vi "G2CPU Line Indexes To Coordinates.vi"(4 "Auto Release Points of Interest on Lines (Enabled)":bool=TRUE, 6 "Auto Release Line Indexers":T1={"Auto Release Line Indexers (Enabled)"=TRUE, "Auto Release Keys (Enabled)"=TRUE}, 8 "error in (no error)":errorcluster, 10 "Line Indexers":T3, 11 "Point of Interest on Lines":refnum<class "1D Array f32.lvclass">) -> (0 "error out":errorcluster, 3 "Coordinates Out":T2)   [LabVIEW 2020, in "G2CPU Line Profile.lvlib"]
doc: "Transform locations on the line profiles to coordinates on the image."
uses:
  G2CPU Line Profile.lvlib
  <vilib>/Natan Biesmans/G2CPU GPU and CPU HPC Toolkit/G2CPU Libraries/Arrays/1DArray/f32/1D Array f32.lvclass
  C:/Program Files/National Instruments/LabVIEW 2025/vi.lib/Natan Biesmans/G2CPU GPU and CPU HPC Toolkit/G2CPU Libraries/Arrays/Array/Array Prototype.lvclass
  <vilib>/Natan Biesmans/G2CPU GPU and CPU HPC Toolkit/G2CPU Libraries/Arrays/2DArray/f32/2D Array f32.lvclass
  <vilib>/Natan Biesmans/G2CPU GPU and CPU HPC Toolkit/G2CPU Libraries/Arrays/2DArray/u32/2D Array u32.lvclass
  <vilib>/Natan Biesmans/G2CPU GPU and CPU HPC Toolkit/G2CPU Libraries/Arrays/1DArray/u32/1D Array u32.lvclass
  <vilib>/Natan Biesmans/G2CPU GPU and CPU HPC Toolkit/G2CPU Libraries/Assignment and indexing/Indexers/G2CPU Indexers.lvclass/G2CPU Indexers.ctl
  <vilib>/Natan Biesmans/G2CPU GPU and CPU HPC Toolkit/G2CPU Libraries/Arrays/Array/Array Prototype.lvclass/Array Prototype.ctl
  6af54969-3e89-456c-a305-a66f3c4e0a45.vi
  a8428e5e-e638-4b8f-97b1-1dfa639c029e.vi
  cd2e55c8-9bfa-4798-9cad-c9068625d012.vi
  0cc7a96f-73a6-40f4-8601-915cc3ecb668.vi
  a76dfa27-2fb7-4ce4-a6bc-f21a5bf6cb57.vi
  af729f83-0425-4644-a175-0b2d98955893.vi
  2fdfb383-b567-4129-8a88-0dd6299b1c5c.vi
  16f8b6bd-ee5f-4b77-ad5a-b16a773401c6.vi
  240874d8-aa58-4a67-9154-73ea1cbf8ba2.vi
  4e0f6f57-f7b3-4ae1-a782-0e163578409f.vi
  bb7fe687-00b1-4455-be70-867d530c61a9.vi
  d411a91c-f4fd-4c23-b328-89003a8b9fa9.vi
  0eb13b9f-5540-4dae-96e9-dbe1488eafb0.vi
  b1fa1afe-a8d8-4705-ab8c-01af7051f9a8.vi
  24612132-8e46-4228-9c8d-2f2d4fc0b450.vi
  a8f317de-a3ee-4dc2-bb18-38ac143a68e4.vi
  788818c2-d318-43e7-b0fc-c88029d63408.vi
  b03dc83b-e216-4518-af22-f4bd8ac76618.vi
  <vilib>/Natan Biesmans/G2CPU GPU and CPU HPC Toolkit/G2CPU Libraries/Assignment and indexing/Indexers/G2CPU Create Indexer.vi
  <vilib>/Natan Biesmans/G2CPU GPU and CPU HPC Toolkit/G2CPU Libraries/Assignment and indexing/Indexers/G2CPU Add Sequencer.vi
  6af54969-3e89-456c-a305-a66f3c4e0a45.vi/4a09c0ae-6cb4-4568-a5ad-7980d18d146b.vi
  6af54969-3e89-456c-a305-a66f3c4e0a45.vi/9f568e59-a541-4346-a017-6cb4bc957f61.vi
  6af54969-3e89-456c-a305-a66f3c4e0a45.vi/c972bab7-bbaf-49da-9265-270ac06aa9b1.vi
  6af54969-3e89-456c-a305-a66f3c4e0a45.vi/693b35e6-7886-4543-b6bf-58b41be5c5ca.vi
  6af54969-3e89-456c-a305-a66f3c4e0a45.vi/9ef54e8b-cde1-4413-ad7f-8efe3ab0591f.vi
  6af54969-3e89-456c-a305-a66f3c4e0a45.vi/d54d4b2e-96c7-4097-8c0a-576c6fb591be.vi
  <vilib>/Natan Biesmans/G2CPU GPU and CPU HPC Toolkit/G2CPU Libraries/Arrays/Array/G2CPU Get Array Pointer.vi
  a8428e5e-e638-4b8f-97b1-1dfa639c029e.vi/cf27cc0d-1fb9-4e2f-ac40-7e8a0db6b27f.vi
  a8428e5e-e638-4b8f-97b1-1dfa639c029e.vi/1874d702-7e82-49f0-9e52-8a9dc00bddc1.vi
  a8428e5e-e638-4b8f-97b1-1dfa639c029e.vi/d603c635-5557-46f9-9702-9944444483a4.vi
  cd2e55c8-9bfa-4798-9cad-c9068625d012.vi/2cbae9c5-d993-4013-91e6-67de96abb5a0.vi
  cd2e55c8-9bfa-4798-9cad-c9068625d012.vi/df7b902d-6356-419a-b5d5-2ac54df1e506.vi
  0cc7a96f-73a6-40f4-8601-915cc3ecb668.vi/6197f869-f6d4-49b3-9b2c-cc979b422c2e.vi
  0cc7a96f-73a6-40f4-8601-915cc3ecb668.vi/a7e86dbb-b4c0-485c-89c5-522e60ee265c.vi
  a76dfa27-2fb7-4ce4-a6bc-f21a5bf6cb57.vi/5793b77b-c002-4ebf-9075-685617c95341.vi
  a76dfa27-2fb7-4ce4-a6bc-f21a5bf6cb57.vi/2ed3ef86-c00d-4d71-b84c-20267a6dfcf9.vi
  af729f83-0425-4644-a175-0b2d98955893.vi/4181b2af-0669-475f-8228-b34a8d51a6f4.vi
  2fdfb383-b567-4129-8a88-0dd6299b1c5c.vi/e7247370-a01f-465a-ac0e-4dfefcb1bb87.vi
  2fdfb383-b567-4129-8a88-0dd6299b1c5c.vi/345e91f0-9a5e-4de4-af9c-133346717e4a.vi
  16f8b6bd-ee5f-4b77-ad5a-b16a773401c6.vi/7467a0f1-0650-4e63-b635-b3d2b2ec9a4e.vi
  16f8b6bd-ee5f-4b77-ad5a-b16a773401c6.vi/8ee11bc3-5ef5-497e-97f0-8db2b3aaa149.vi
  16f8b6bd-ee5f-4b77-ad5a-b16a773401c6.vi/c7af9698-5e3c-4e11-95da-3024075b67d2.vi
  240874d8-aa58-4a67-9154-73ea1cbf8ba2.vi/2e03f477-51b7-4ba0-bb4f-4f838f6557e6.vi
  240874d8-aa58-4a67-9154-73ea1cbf8ba2.vi/125d45d4-836b-469d-8a4a-6adb452f866d.vi
  240874d8-aa58-4a67-9154-73ea1cbf8ba2.vi/8038e9ed-2e71-4568-91ba-0d873494c5ed.vi
  4e0f6f57-f7b3-4ae1-a782-0e163578409f.vi/9d769ba4-bbb4-4eb6-9175-95d7d139327c.vi
  4e0f6f57-f7b3-4ae1-a782-0e163578409f.vi/8bfea9e7-a130-4d69-b32e-15c58d17157f.vi
  4e0f6f57-f7b3-4ae1-a782-0e163578409f.vi/25f1b8bb-c437-45f4-b6eb-f3e32cc20aa5.vi
  4e0f6f57-f7b3-4ae1-a782-0e163578409f.vi/309f54b5-9a40-4a1d-900d-2d620fefb202.vi
  bb7fe687-00b1-4455-be70-867d530c61a9.vi/bb516b05-0a1d-45df-9cb0-c772dcc1833e.vi
  bb7fe687-00b1-4455-be70-867d530c61a9.vi/2071ba82-ee09-44c2-9784-3e752811cb07.vi
  bb7fe687-00b1-4455-be70-867d530c61a9.vi/c68a08d6-cad3-47fe-810c-4c138e8e5bf7.vi
  bb7fe687-00b1-4455-be70-867d530c61a9.vi/599fcc89-82aa-4e20-b9df-949478d910a7.vi
  d411a91c-f4fd-4c23-b328-89003a8b9fa9.vi/ce577589-e75d-42be-a3c5-f5395febe2a6.vi
  d411a91c-f4fd-4c23-b328-89003a8b9fa9.vi/d13051aa-bce5-446f-b44f-e7ab7cfb1f03.vi
  d411a91c-f4fd-4c23-b328-89003a8b9fa9.vi/ca2a5711-2ea0-41ce-865a-169a0e3bc9ca.vi
  0eb13b9f-5540-4dae-96e9-dbe1488eafb0.vi/f4654d05-beb0-4753-bab7-24376daae318.vi
  0eb13b9f-5540-4dae-96e9-dbe1488eafb0.vi/a2f9e1c9-c94e-4cd6-9432-cf54c3ac582a.vi
  b1fa1afe-a8d8-4705-ab8c-01af7051f9a8.vi/d8f9d983-4edf-44a2-8364-f00f0b470774.vi
  b1fa1afe-a8d8-4705-ab8c-01af7051f9a8.vi/83167447-a0f5-45d9-a71d-4def8f50970d.vi
  24612132-8e46-4228-9c8d-2f2d4fc0b450.vi/cfed8f62-9c64-4dab-912e-5e7c21cb720b.vi
  a8f317de-a3ee-4dc2-bb18-38ac143a68e4.vi/d8f9d983-4edf-44a2-8364-f00f0b470774.vi
  a8f317de-a3ee-4dc2-bb18-38ac143a68e4.vi/83167447-a0f5-45d9-a71d-4def8f50970d.vi
  788818c2-d318-43e7-b0fc-c88029d63408.vi/cfed8f62-9c64-4dab-912e-5e7c21cb720b.vi
  b03dc83b-e216-4518-af22-f4bd8ac76618.vi/d8f9d983-4edf-44a2-8364-f00f0b470774.vi
  b03dc83b-e216-4518-af22-f4bd8ac76618.vi/83167447-a0f5-45d9-a71d-4def8f50970d.vi
  <vilib>/Natan Biesmans/G2CPU GPU and CPU HPC Toolkit/G2CPU Libraries/Assignment and indexing/Indexers/G2CPU Get indexers Pointer.vi
  a8428e5e-e638-4b8f-97b1-1dfa639c029e.vi/cf27cc0d-1fb9-4e2f-ac40-7e8a0db6b27f.vi/3e802c67-fb96-46a3-ae13-4994a8508b4f.vi
  a8428e5e-e638-4b8f-97b1-1dfa639c029e.vi/cf27cc0d-1fb9-4e2f-ac40-7e8a0db6b27f.vi/5a50fc67-79e7-4972-80c2-92243cd53dd4.vi
  a8428e5e-e638-4b8f-97b1-1dfa639c029e.vi/cf27cc0d-1fb9-4e2f-ac40-7e8a0db6b27f.vi/4b7910ad-0c4a-46e4-b1b3-c9721aeaa91e.vi
  a8428e5e-e638-4b8f-97b1-1dfa639c029e.vi/1874d702-7e82-49f0-9e52-8a9dc00bddc1.vi/77c7badc-ed81-4514-99c1-20d37f4e5ecc.vi
  a8428e5e-e638-4b8f-97b1-1dfa639c029e.vi/1874d702-7e82-49f0-9e52-8a9dc00bddc1.vi/eb76fa01-6782-47b4-b34f-9eb474c9cc78.vi
  <vilib>/Natan Biesmans/G2CPU GPU and CPU HPC Toolkit/ArrayFire Driver/VIs/Run as Multi Device.vi
  a8428e5e-e638-4b8f-97b1-1dfa639c029e.vi/d603c635-5557-46f9-9702-9944444483a4.vi/730f6c57-5c0b-4ee9-b61e-75067b25222b.vi
  a8428e5e-e638-4b8f-97b1-1dfa639c029e.vi/d603c635-5557-46f9-9702-9944444483a4.vi/096b8799-7810-404e-baca-ba9279cec4bd.vi
  a8428e5e-e638-4b8f-97b1-1dfa639c029e.vi/d603c635-5557-46f9-9702-9944444483a4.vi/0f1a5a47-bcc5-4796-ac31-8dfcfbc0d7d1.vi
  a8428e5e-e638-4b8f-97b1-1dfa639c029e.vi/d603c635-5557-46f9-9702-9944444483a4.vi/89f12e17-3330-4b72-ad8f-8dd636660732.vi
  cd2e55c8-9bfa-4798-9cad-c9068625d012.vi/df7b902d-6356-419a-b5d5-2ac54df1e506.vi/6058dca8-195d-4566-b47b-6d6a1c5af61f.vi
  0cc7a96f-73a6-40f4-8601-915cc3ecb668.vi/6197f869-f6d4-49b3-9b2c-cc979b422c2e.vi/3e802c67-fb96-46a3-ae13-4994a8508b4f.vi
  0cc7a96f-73a6-40f4-8601-915cc3ecb668.vi/6197f869-f6d4-49b3-9b2c-cc979b422c2e.vi/5a50fc67-79e7-4972-80c2-92243cd53dd4.vi
  0cc7a96f-73a6-40f4-8601-915cc3ecb668.vi/6197f869-f6d4-49b3-9b2c-cc979b422c2e.vi/4b7910ad-0c4a-46e4-b1b3-c9721aeaa91e.vi
  0cc7a96f-73a6-40f4-8601-915cc3ecb668.vi/a7e86dbb-b4c0-485c-89c5-522e60ee265c.vi/730f6c57-5c0b-4ee9-b61e-75067b25222b.vi
  0cc7a96f-73a6-40f4-8601-915cc3ecb668.vi/a7e86dbb-b4c0-485c-89c5-522e60ee265c.vi/096b8799-7810-404e-baca-ba9279cec4bd.vi
  0cc7a96f-73a6-40f4-8601-915cc3ecb668.vi/a7e86dbb-b4c0-485c-89c5-522e60ee265c.vi/0f1a5a47-bcc5-4796-ac31-8dfcfbc0d7d1.vi
  0cc7a96f-73a6-40f4-8601-915cc3ecb668.vi/a7e86dbb-b4c0-485c-89c5-522e60ee265c.vi/89f12e17-3330-4b72-ad8f-8dd636660732.vi
  a76dfa27-2fb7-4ce4-a6bc-f21a5bf6cb57.vi/5793b77b-c002-4ebf-9075-685617c95341.vi/3e802c67-fb96-46a3-ae13-4994a8508b4f.vi
  a76dfa27-2fb7-4ce4-a6bc-f21a5bf6cb57.vi/5793b77b-c002-4ebf-9075-685617c95341.vi/5a50fc67-79e7-4972-80c2-92243cd53dd4.vi
  a76dfa27-2fb7-4ce4-a6bc-f21a5bf6cb57.vi/2ed3ef86-c00d-4d71-b84c-20267a6dfcf9.vi/730f6c57-5c0b-4ee9-b61e-75067b25222b.vi
  a76dfa27-2fb7-4ce4-a6bc-f21a5bf6cb57.vi/2ed3ef86-c00d-4d71-b84c-20267a6dfcf9.vi/096b8799-7810-404e-baca-ba9279cec4bd.vi
  a76dfa27-2fb7-4ce4-a6bc-f21a5bf6cb57.vi/2ed3ef86-c00d-4d71-b84c-20267a6dfcf9.vi/0f1a5a47-bcc5-4796-ac31-8dfcfbc0d7d1.vi
  a76dfa27-2fb7-4ce4-a6bc-f21a5bf6cb57.vi/2ed3ef86-c00d-4d71-b84c-20267a6dfcf9.vi/89f12e17-3330-4b72-ad8f-8dd636660732.vi
  240874d8-aa58-4a67-9154-73ea1cbf8ba2.vi/2e03f477-51b7-4ba0-bb4f-4f838f6557e6.vi/d8e2d9cc-c923-495e-b121-b6b84788c73f.vi
  240874d8-aa58-4a67-9154-73ea1cbf8ba2.vi/2e03f477-51b7-4ba0-bb4f-4f838f6557e6.vi/345e91f0-9a5e-4de4-af9c-133346717e4a.vi
  4e0f6f57-f7b3-4ae1-a782-0e163578409f.vi/8bfea9e7-a130-4d69-b32e-15c58d17157f.vi/6058dca8-195d-4566-b47b-6d6a1c5af61f.vi
  4e0f6f57-f7b3-4ae1-a782-0e163578409f.vi/309f54b5-9a40-4a1d-900d-2d620fefb202.vi/730f6c57-5c0b-4ee9-b61e-75067b25222b.vi
  4e0f6f57-f7b3-4ae1-a782-0e163578409f.vi/309f54b5-9a40-4a1d-900d-2d620fefb202.vi/096b8799-7810-404e-baca-ba9279cec4bd.vi
  4e0f6f57-f7b3-4ae1-a782-0e163578409f.vi/309f54b5-9a40-4a1d-900d-2d620fefb202.vi/0f1a5a47-bcc5-4796-ac31-8dfcfbc0d7d1.vi
  4e0f6f57-f7b3-4ae1-a782-0e163578409f.vi/309f54b5-9a40-4a1d-900d-2d620fefb202.vi/89f12e17-3330-4b72-ad8f-8dd636660732.vi
  bb7fe687-00b1-4455-be70-867d530c61a9.vi/bb516b05-0a1d-45df-9cb0-c772dcc1833e.vi/46771f49-eb1d-473b-8e81-f516cef50a4e.vi
  bb7fe687-00b1-4455-be70-867d530c61a9.vi/bb516b05-0a1d-45df-9cb0-c772dcc1833e.vi/dc76f8e4-64fa-456a-8549-7a4b6936c4c9.vi
  bb7fe687-00b1-4455-be70-867d530c61a9.vi/bb516b05-0a1d-45df-9cb0-c772dcc1833e.vi/7e60ddfb-e748-4c0c-85da-e395a1b7978d.vi
  bb7fe687-00b1-4455-be70-867d530c61a9.vi/bb516b05-0a1d-45df-9cb0-c772dcc1833e.vi/d2eceff7-f641-4ce4-acfa-e9e293a3c877.vi
  bb7fe687-00b1-4455-be70-867d530c61a9.vi/bb516b05-0a1d-45df-9cb0-c772dcc1833e.vi/b737122b-4036-448b-abd3-e2701355e828.vi
  bb7fe687-00b1-4455-be70-867d530c61a9.vi/2071ba82-ee09-44c2-9784-3e752811cb07.vi/a578f522-3460-4434-be98-bad896664269.vi
  bb7fe687-00b1-4455-be70-867d530c61a9.vi/c68a08d6-cad3-47fe-810c-4c138e8e5bf7.vi/e7247370-a01f-465a-ac0e-4dfefcb1bb87.vi
  bb7fe687-00b1-4455-be70-867d530c61a9.vi/c68a08d6-cad3-47fe-810c-4c138e8e5bf7.vi/345e91f0-9a5e-4de4-af9c-133346717e4a.vi
  d411a91c-f4fd-4c23-b328-89003a8b9fa9.vi/d13051aa-bce5-446f-b44f-e7ab7cfb1f03.vi/e7247370-a01f-465a-ac0e-4dfefcb1bb87.vi
  d411a91c-f4fd-4c23-b328-89003a8b9fa9.vi/d13051aa-bce5-446f-b44f-e7ab7cfb1f03.vi/345e91f0-9a5e-4de4-af9c-133346717e4a.vi
  24612132-8e46-4228-9c8d-2f2d4fc0b450.vi/cfed8f62-9c64-4dab-912e-5e7c21cb720b.vi/77c7badc-ed81-4514-99c1-20d37f4e5ecc.vi
  24612132-8e46-4228-9c8d-2f2d4fc0b450.vi/cfed8f62-9c64-4dab-912e-5e7c21cb720b.vi/eb76fa01-6782-47b4-b34f-9eb474c9cc78.vi
  788818c2-d318-43e7-b0fc-c88029d63408.vi/cfed8f62-9c64-4dab-912e-5e7c21cb720b.vi/77c7badc-ed81-4514-99c1-20d37f4e5ecc.vi
  788818c2-d318-43e7-b0fc-c88029d63408.vi/cfed8f62-9c64-4dab-912e-5e7c21cb720b.vi/eb76fa01-6782-47b4-b34f-9eb474c9cc78.vi
  a8428e5e-e638-4b8f-97b1-1dfa639c029e.vi/cf27cc0d-1fb9-4e2f-ac40-7e8a0db6b27f.vi/5a50fc67-79e7-4972-80c2-92243cd53dd4.vi/1b7cf390-2ae0-48f3-9bce-03c57eed6ee8.vi
  cd2e55c8-9bfa-4798-9cad-c9068625d012.vi/df7b902d-6356-419a-b5d5-2ac54df1e506.vi/6058dca8-195d-4566-b47b-6d6a1c5af61f.vi/77c7badc-ed81-4514-99c1-20d37f4e5ecc.vi
  cd2e55c8-9bfa-4798-9cad-c9068625d012.vi/df7b902d-6356-419a-b5d5-2ac54df1e506.vi/6058dca8-195d-4566-b47b-6d6a1c5af61f.vi/eb76fa01-6782-47b4-b34f-9eb474c9cc78.vi
  0cc7a96f-73a6-40f4-8601-915cc3ecb668.vi/6197f869-f6d4-49b3-9b2c-cc979b422c2e.vi/5a50fc67-79e7-4972-80c2-92243cd53dd4.vi/1b7cf390-2ae0-48f3-9bce-03c57eed6ee8.vi
  4e0f6f57-f7b3-4ae1-a782-0e163578409f.vi/8bfea9e7-a130-4d69-b32e-15c58d17157f.vi/6058dca8-195d-4566-b47b-6d6a1c5af61f.vi/77c7badc-ed81-4514-99c1-20d37f4e5ecc.vi
  4e0f6f57-f7b3-4ae1-a782-0e163578409f.vi/8bfea9e7-a130-4d69-b32e-15c58d17157f.vi/6058dca8-195d-4566-b47b-6d6a1c5af61f.vi/eb76fa01-6782-47b4-b34f-9eb474c9cc78.vi
  bb7fe687-00b1-4455-be70-867d530c61a9.vi/bb516b05-0a1d-45df-9cb0-c772dcc1833e.vi/dc76f8e4-64fa-456a-8549-7a4b6936c4c9.vi/3e802c67-fb96-46a3-ae13-4994a8508b4f.vi
  bb7fe687-00b1-4455-be70-867d530c61a9.vi/bb516b05-0a1d-45df-9cb0-c772dcc1833e.vi/dc76f8e4-64fa-456a-8549-7a4b6936c4c9.vi/5a50fc67-79e7-4972-80c2-92243cd53dd4.vi
  bb7fe687-00b1-4455-be70-867d530c61a9.vi/bb516b05-0a1d-45df-9cb0-c772dcc1833e.vi/dc76f8e4-64fa-456a-8549-7a4b6936c4c9.vi/4b7910ad-0c4a-46e4-b1b3-c9721aeaa91e.vi
  bb7fe687-00b1-4455-be70-867d530c61a9.vi/bb516b05-0a1d-45df-9cb0-c772dcc1833e.vi/dc76f8e4-64fa-456a-8549-7a4b6936c4c9.vi/5a50fc67-79e7-4972-80c2-92243cd53dd4.vi/1b7cf390-2ae0-48f3-9bce-03c57eed6ee8.vi
  <vilib>/Natan Biesmans/G2CPU GPU and CPU HPC Toolkit/G2CPU Libraries/Arrays/1DArray/binary/1D Array binary.lvclass
  <vilib>/Natan Biesmans/G2CPU GPU and CPU HPC Toolkit/G2CPU Libraries/Arrays/1DArray/s32/1D Array s32.lvclass
  <vilib>/Natan Biesmans/G2CPU GPU and CPU HPC Toolkit/ArrayFire Driver/VIs/create indexers.vi
  <vilib>/Natan Biesmans/G2CPU GPU and CPU HPC Toolkit/ArrayFire Driver/VIs/set seq param indexer.vi
  <vilib>/Natan Biesmans/G2CPU GPU and CPU HPC Toolkit/ArrayFire Driver/VIs/index gen.vi
  <vilib>/Natan Biesmans/G2CPU GPU and CPU HPC Toolkit/ArrayFire Driver/VIs/get dims.vi
  <vilib>/Natan Biesmans/G2CPU GPU and CPU HPC Toolkit/G2CPU Libraries/Assignment and indexing/Indexers/IndexedDimsToDimCluster.vi
  <vilib>/Natan Biesmans/G2CPU GPU and CPU HPC Toolkit/ArrayFire Driver/VIs/reorder.vi
  <vilib>/Natan Biesmans/G2CPU GPU and CPU HPC Toolkit/ArrayFire Driver/VIs/release array.vi
  <vilib>/Natan Biesmans/G2CPU GPU and CPU HPC Toolkit/G2CPU Libraries/Arrays/Array/G2CPU Set Array Pointer.vi
  <vilib>/Natan Biesmans/G2CPU GPU and CPU HPC Toolkit/G2CPU Libraries/Assignment and indexing/Indexers/G2CPU Release Indexer.vi
  <vilib>/Natan Biesmans/G2CPU GPU and CPU HPC Toolkit/G2CPU Libraries/Arrays/Array/G2CPU Release Array.vi
  <vilib>/Natan Biesmans/G2CPU GPU and CPU HPC Toolkit/ArrayFire Driver/VIs/iszero.vi
  <vilib>/Natan Biesmans/G2CPU GPU and CPU HPC Toolkit/ArrayFire Driver/VIs/sub.vi
  <vilib>/Natan Biesmans/G2CPU GPU and CPU HPC Toolkit/ArrayFire Driver/subvi/Error Converter (ErrCode or Status).vi
  <vilib>/Natan Biesmans/G2CPU GPU and CPU HPC Toolkit/ArrayFire Driver/VIs/cast.vi
  <vilib>/Natan Biesmans/G2CPU GPU and CPU HPC Toolkit/ArrayFire Driver/VIs/add.vi
  <vilib>/Natan Biesmans/G2CPU GPU and CPU HPC Toolkit/ArrayFire Driver/VIs/accum.vi
  <vilib>/Natan Biesmans/G2CPU GPU and CPU HPC Toolkit/G2CPU Libraries/Arrays/SubVI/RemoveReducedDimensionForReorder.vi
  <vilib>/Natan Biesmans/G2CPU GPU and CPU HPC Toolkit/G2CPU Libraries/Arrays/SubVI/is 1D.vi
  <vilib>/Natan Biesmans/G2CPU GPU and CPU HPC Toolkit/ArrayFire Driver/VIs/lt.vi
  <vilib>/Natan Biesmans/G2CPU GPU and CPU HPC Toolkit/ArrayFire Driver/VIs/mul.vi
  <vilib>/Natan Biesmans/G2CPU GPU and CPU HPC Toolkit/ArrayFire Driver/VIs/round.vi
  <vilib>/Natan Biesmans/G2CPU GPU and CPU HPC Toolkit/ArrayFire Driver/VIs/flat.vi
  <vilib>/Natan Biesmans/G2CPU GPU and CPU HPC Toolkit/ArrayFire Driver/VIs/lookup.vi
  <vilib>/Natan Biesmans/G2CPU GPU and CPU HPC Toolkit/ArrayFire Driver/VIs/mod.vi
  <vilib>/Natan Biesmans/G2CPU GPU and CPU HPC Toolkit/ArrayFire Driver/VIs/div.vi
  <vilib>/Natan Biesmans/G2CPU GPU and CPU HPC Toolkit/ArrayFire Driver/VIs/trunc.vi
  <vilib>/Natan Biesmans/G2CPU GPU and CPU HPC Toolkit/ArrayFire Driver/VIs/sign.vi
  <vilib>/Natan Biesmans/G2CPU GPU and CPU HPC Toolkit/ArrayFire Driver/VIs/not.vi
  <vilib>/Natan Biesmans/G2CPU GPU and CPU HPC Toolkit/ArrayFire Driver/VIs/replace.vi
  <vilib>/Natan Biesmans/G2CPU GPU and CPU HPC Toolkit/G2CPU Libraries/Arrays/Array/Array Prototype.lvclass
  <vilib>/Natan Biesmans/G2CPU GPU and CPU HPC Toolkit/G2CPU Libraries/Assignment and indexing/Indexers/G2CPU Indexers.lvclass
  <vilib>/Natan Biesmans/G2CPU GPU and CPU HPC Toolkit/G2CPU Libraries/Arrays/DataTypes/U32/U32.lvclass
  <vilib>/Natan Biesmans/G2CPU GPU and CPU HPC Toolkit/G2CPU Libraries/Arrays/2DArray/2D Array Prototype.lvclass
  <vilib>/Natan Biesmans/G2CPU GPU and CPU HPC Toolkit/G2CPU Libraries/Arrays/1DArray/1D Array Prototype.lvclass
  <vilib>/Natan Biesmans/G2CPU GPU and CPU HPC Toolkit/G2CPU Libraries/Arrays/DataTypes/f32/f32.lvclass
  <vilib>/Natan Biesmans/G2CPU GPU and CPU HPC Toolkit/G2CPU Libraries/Arrays/DataTypes/I32/s32.lvclass
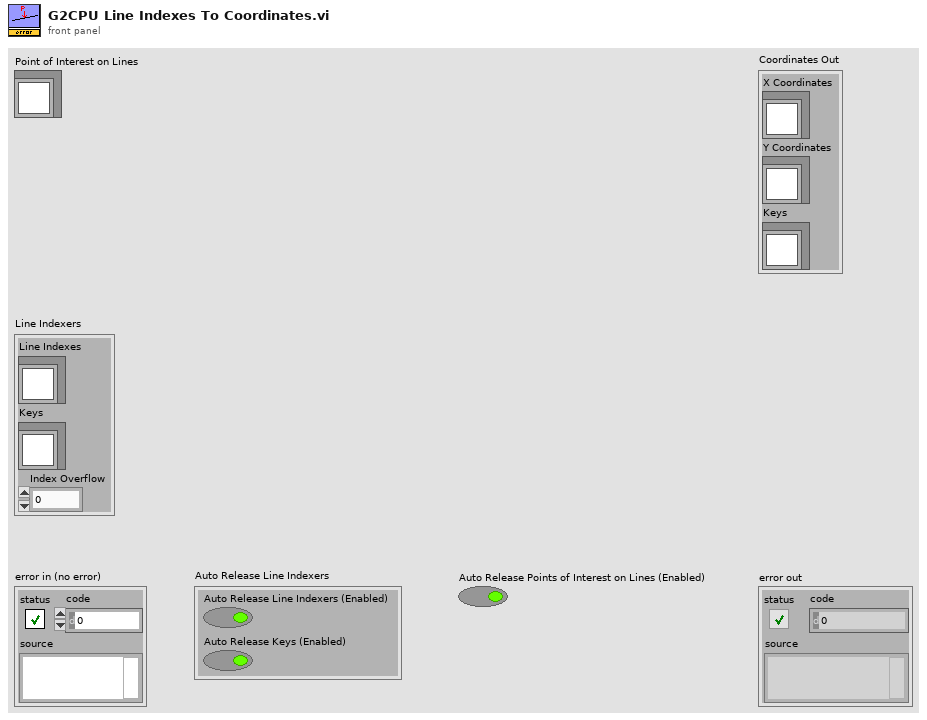
[diagram p1: front panel]
types:
  T1 = cluster{"Auto Release Line Indexers (Enabled)":bool, "Auto Release Keys (Enabled)":bool}
  T2 = cluster{"X Coordinates":refnum<class "1D Array f32.lvclass">, "Y Coordinates":refnum<class "1D Array f32.lvclass">, "Keys":refnum<class "1D Array u32.lvclass">}
  T3 = cluster{"Line Indexes":refnum<class "2D Array f32.lvclass">, "Keys":refnum<class "2D Array u32.lvclass">, "Index Overflow":u64}
  T4 = cluster{"Y Coordinates":refnum<class "1D Array f32.lvclass">, "X Coordinates":refnum<class "1D Array f32.lvclass">, "Keys":refnum<class "1D Array u32.lvclass">}
  T5 = typedef "AF.lvlib/Dim4.ctl" = cluster{"Dim 0":u64, "Dim 1":u64, "Dim 2":u64, "Dim 3":u64}
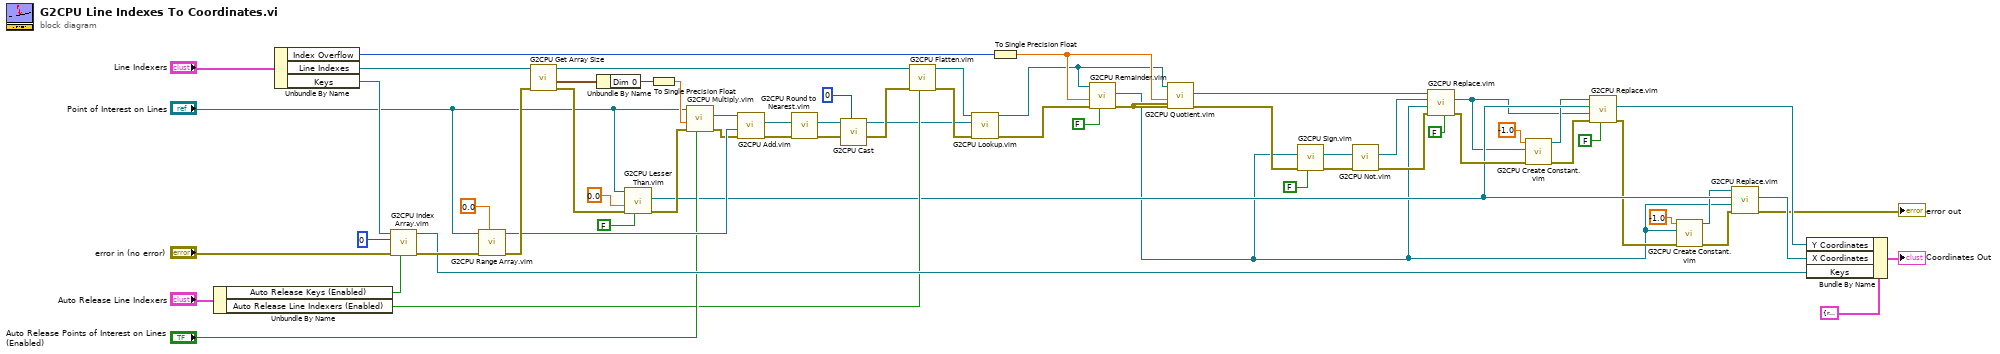
[diagram p0: block diagram]
diagram:
  n1 = Unbundle By Name("Auto Release Line Indexers") -> ("Auto Release Keys (Enabled)"=w32:bool, "Auto Release Line Indexers (Enabled)"=w31:bool)
  n2 = Unbundle By Name("Line Indexers") -> ("Index Overflow"=w62:u64, "Line Indexes"=w41:refnum<class "2D Array f32.lvclass">, "Keys"=w38:refnum<class "2D Array u32.lvclass">)
  n3 = call "G2CPU Index Array.vim"("Auto Release Array In (Enabled)"=w32, "error in (no error)"="error in (no error)", "Indexes"=0, "Array In"=w38) -> ("error out"=w37:errorcluster, "Array Index"=w35:refnum<class "1D Array u32.lvclass">)  [unwired: 6 in]
  n4 = call "G2CPU Range Array.vim"("Datatype"=sgl 0.0, "Error in"=w37, "Size"="Point of Interest on Lines") -> ("error out"=w64:errorcluster, "Array out"=w54:refnum<class "1D Array f32.lvclass">)  [unwired: 7 in]
  n5 = call <vilib>:"G2CPU Get Array Size.vi"("error in (no error)"=w64, "Array in"=w41) -> ("error out"=w18:errorcluster, "Array Size"=w65:T5, "Array out"=w57:refnum<class "2D Array f32.lvclass">)  [unwired: 6 in, 1 out]
  n6 = Unbundle By Name(w65) -> ("Dim 0"=w59:u64)
  n7 = call "G2CPU Lesser Than.vim"("Auto Release lhs (Enabled)"=FALSE ("Auto Release rhs (Enabled)"), "error in (no error)"=w18, "Array rhs"=sgl 0.0, "Array lhs"="Point of Interest on Lines") -> ("error out"=w17:errorcluster, "Array Result"=w10:refnum<class "1D Array binary.lvclass">)  [unwired: 6 in]
  n8 = To Single Precision Float(number=w59) -> (single precision float=w56:sgl)
  n9 = call "G2CPU Multiply.vim"("Auto Release lhs"="Auto Release Points of Interest on Lines (Enabled)", "error in (no error)"=w17, "Array rhs"=w56, "Array lhs"="Point of Interest on Lines") -> ("error out"=w53:errorcluster, "Array Result"=w55:refnum<class "1D Array f32.lvclass">)  [unwired: 6 in]
  n10 = call "G2CPU Add.vim"("error in (no error)"=w53, "Array rhs"=w54, "Array lhs"=w55) -> ("error out"=w27:errorcluster, "Array Result"=w26:refnum<class "1D Array f32.lvclass">)  [unwired: 7 in]
  n11 = call "G2CPU Round to Nearest.vim"("error in (no error)"=w27, "Array in"=w26) -> ("error out"=w24:errorcluster, "Array Result"=w25:refnum<class "1D Array f32.lvclass">)  [unwired: 8 in]
  n12 = call "G2CPU Cast"("Datatype Prototype"=u32 0, "error in (no error)"=w24, "Array In"=w25) -> ("error out"=w23:errorcluster, "Array Out"=w21:refnum<class "1D Array u32.lvclass">)  [unwired: 7 in]
  n13 = call "G2CPU Flatten.vim"("Auto Release (Enabled)"=w31, "error in (no error)"=w23, "Array In"=w57) -> ("error out"=w46:errorcluster, "Array out"=w45:refnum<class "1D Array f32.lvclass">)  [unwired: 7 in]
  n14 = call "G2CPU Lookup.vim"("error in (no error)"=w46, "Indices (1D)"=w21, "Array In"=w45) -> ("error out"=w44:errorcluster, "Indexed Array"=w43:refnum<class "1D Array f32.lvclass">)  [unwired: 7 in]
  n15 = To Single Precision Float(number=w62) -> (single precision float=w60:sgl)
  n16 = call "G2CPU Remainder.vim"("Auto Release lhs (Enabled)"=FALSE, "error in (no error)"=w44, "Array rhs"=w60, "Array lhs"=w43) -> ("error out"=w28:errorcluster, "Array Result"=w1:refnum<class "1D Array f32.lvclass">)  [unwired: 6 in]
  n17 = call "G2CPU Quotient.vim"("Auto Release lhs (Enabled)"=w28, "error in (no error)"=w28, "Array rhs"=w60, "Array lhs"=w43) -> ("error out"=w58:errorcluster, "Array Result"=w29:refnum<class "1D Array f32.lvclass">)  [unwired: 6 in]
  n18 = call "G2CPU Sign.vim"("Auto Release (Enabled)"=FALSE, "error in (no error)"=w58, "Array in"=w1) -> ("error out"=w47:errorcluster, "Array Result"=w48:refnum<class "1D Array binary.lvclass">)  [unwired: 7 in]
  n19 = call "G2CPU Not.vim"("error in (no error)"=w47, "Array in"=w48) -> ("error out"=w50:errorcluster, "Array Result"=w51:refnum<class "1D Array binary.lvclass">)  [unwired: 8 in]
  n20 = call "G2CPU Replace.vim"("Auto Release Replace Values (Enabled)"=FALSE, "error in (no error)"=w50, "To Replace Values Array or scalar Value"=w1, "Replace  Condition"=w51, "Array In"=w29) -> ("error out"=w13:errorcluster, "Array out (same as in)"=w3:refnum<class "1D Array f32.lvclass">)  [unwired: 5 in]
  n21 = call "G2CPU Create Constant.vim"("error in (no error)"=w13, "Size"=w3, "val"=sgl -1.0) -> ("error out"=w15:errorcluster, "object out"=w4:refnum<class "1D Array f32.lvclass">)  [unwired: 7 in]
  n22 = call "G2CPU Replace.vim"("Auto Release Replace Condition (Enabled)"=FALSE, "error in (no error)"=w15, "To Replace Values Array or scalar Value"=w3, "Replace  Condition"=w10, "Array In"=w4) -> ("error out"=w8:errorcluster, "Array out (same as in)"=w11:refnum<class "1D Array f32.lvclass">)  [unwired: 5 in]
  n23 = call "G2CPU Create Constant.vim"("error in (no error)"=w8, "Size"=w1, "val"=sgl -1.0) -> ("error out"=w7:errorcluster, "object out"=w2:refnum<class "1D Array f32.lvclass">)  [unwired: 7 in]
  n24 = call "G2CPU Replace.vim"("error in (no error)"=w7, "To Replace Values Array or scalar Value"=w1, "Replace  Condition"=w10, "Array In"=w2) -> ("error out"=→"error out":errorcluster, "Array out (same as in)"=w6:refnum<class "1D Array f32.lvclass">)  [unwired: 6 in]
  n25 = Bundle By Name(cluster=T4 {"Y Coordinates"=refnum, "X Coordinates"=refnum, "Keys"=refnum} ("Coordinates Out"), "Y Coordinates"=w11, "X Coordinates"=w6, "Keys"=w35) -> (→"Coordinates Out":T4)
